vi "get version info.vi"(8 "error in":errorcluster) -> (0 "error out":errorcluster, 2 "FileVersion":string, 3 "Title":string)   [LabVIEW 2023]
doc: "This VI will return the Version info of the exe during runtime environment."
panel:
  in  "Date":string=" Build Date: 09-Jan-2025 "
  # "VI Template By\n        Samuel James\n        Measurement Engineer\n        Certified LabVIEW Architect\n        Vestas Technology R&D Chennai"
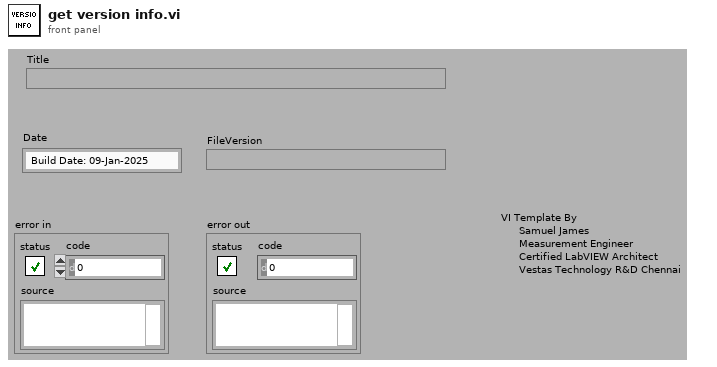
[diagram p1: front panel]
types:
  T1 = enum32{"invalid app kind", "Development System", "Run Time System", "Student Edition", "Embedded LabVIEW", "Evaluation", "Custom"}
  T2 = cluster{"Major":i32, "Minor":i32, "Micro":i32, "Build":i32}
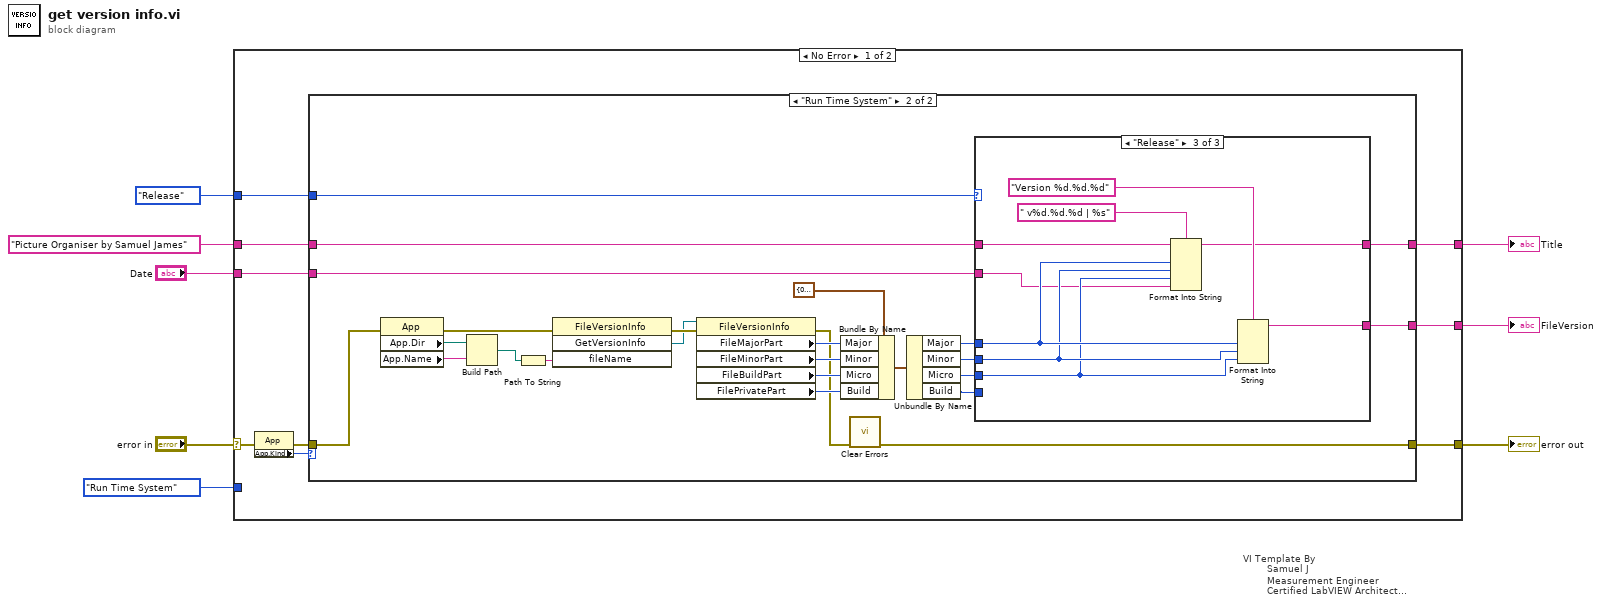
[diagram p0: block diagram]
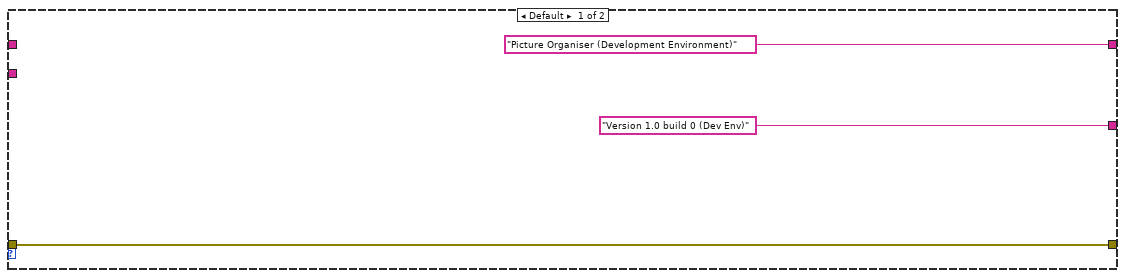
[diagram p2: hidden frame]
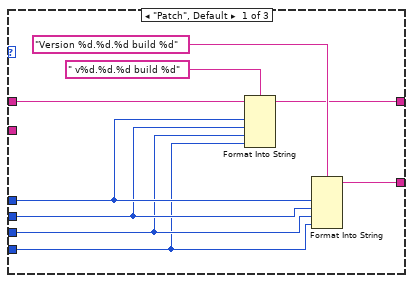
[diagram p3: hidden frame]
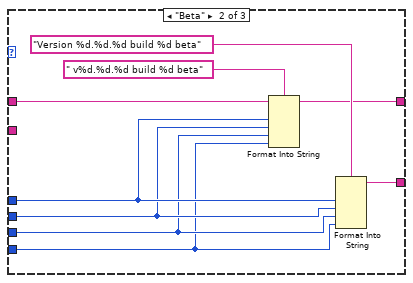
[diagram p4: hidden frame]
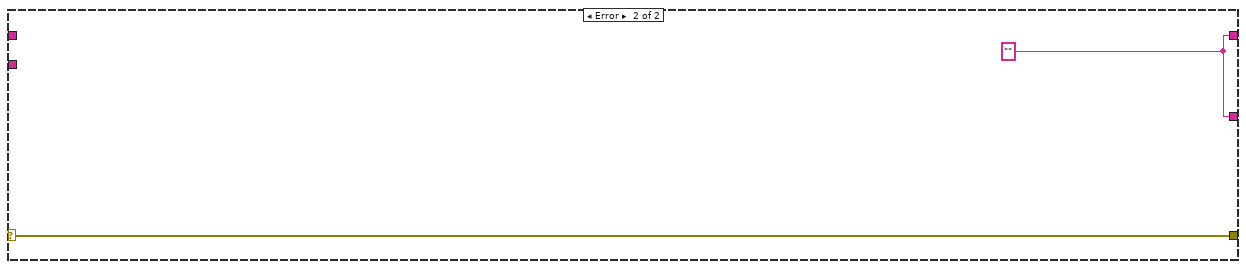
[diagram p5: hidden frame]
diagram:
  n1 = case "VI Template By\n        Samuel J\n        Measurement Engineer\n        Certified LabVIEW Architect\n        Vestas Technology R&D, Chennai" shown="No Error" "error in" {
    selector: "error in" -> [w12 w74]
    tunnel: [w17 w73] -> w8
    tunnel: [w16 w74] -> w6
    tunnel: [w14 w73] -> w5
    tunnel: "Picture Organiser by Samuel James" ("Product Name") -> [w13 _]
    tunnel: T1."Run Time System" ("App.Kind") -> [_ _]
    tunnel: enum16{"Release", "Patch", "Beta"}."Release" -> [w11 _]
    tunnel: "Date" -> [w10 _]
    frame No Error {
      n2 = property class="App"(error in=w12) -> (error out=w15:errorcluster, "App.Kind"=w9:T1)  [unwired: 1 in, 1 out]
      n3 = case shown="\"Run Time System\"" w9 {
        tunnel: ["Version 1.0 build 0 (Dev Env)" w45] -> w17
        tunnel: [w20 w23] -> w16
        tunnel: w15 -> [w20 w42]
        tunnel: ["Picture Organiser (Development Environment)" w44] -> w14
        tunnel: w13 -> [_ w43]
        tunnel: w11 -> [_ w29]
        tunnel: w10 -> [_ w22]
        frame Default {
        }
        frame "Run Time System" {
          n4 = property class="App"(error in=w42) -> (error out=w41:errorcluster, "App.Dir"=w36:path, "App.Name"=w37:string)  [unwired: 1 in, 1 out]
          n5 = Build Path(base path=w36, name or relative path=w37) -> (appended path=w21:path)
          n6 = Path To String(path=w21) -> (string=w40:string)
          n7 = invoke class="FileVersionInfo" method="GetVersionInfo"(error in=w41, "fileName"=w40) -> (error out=w39:errorcluster, "GetVersionInfo"=w38:refnum<k24>)  [unwired: 2 in, 2 out]
          n8 = property class="FileVersionInfo"(reference=w38, error in=w39) -> (error out=w30:errorcluster, "FileMajorPart"=w34:i32, "FileMinorPart"=w33:i32, "FileBuildPart"=w32:i32, "FilePrivatePart"=w31:i32)  [unwired: 1 out]
          n9 = Bundle By Name(cluster=T2 {"Major"=0, "Minor"=0, "Micro"=0, "Build"=0} ("Cluster"), "Major"=w34, "Minor"=w33, "Micro"=w32, "Build"=w31) -> (w28:T2)
          n10 = call <vilib>:"Clear Errors.vi"("error in (no error)"=w30) -> ("error out"=w23:errorcluster)  [unwired: 5 in, 1 out]
          n11 = Unbundle By Name(w28) -> ("Major"=w27:i32, "Minor"=w26:i32, "Micro"=w25:i32, "Build"=w24:i32)
          n12 = case shown="\"Release\"" w29 {
            tunnel: [w53 w62 w71] -> w45
            tunnel: [w51 w60 w69] -> w44
            tunnel: w43 -> [w50 w59 w68]
            tunnel: w27 -> [w49 w58 w67]
            tunnel: w26 -> [w48 w57 w66]
            tunnel: w25 -> [w47 w56 w65]
            tunnel: w24 -> [w46 w55 _]
            tunnel: w22 -> [_ _ w64]
            frame "Patch", Default {
              n13 = Format Into String(format string=" v%d.%d.%d build %d", initial string=w50, w49, w48, w47, w46) -> (resulting string=w51:string)  [unwired: 1 in, 1 out]
              n14 = Format Into String(format string="Version %d.%d.%d build %d", w49, w48, w47, w46) -> (resulting string=w53:string)  [unwired: 2 in, 1 out]
            }
            frame "Beta" {
              n15 = Format Into String(format string=" v%d.%d.%d build %d beta", initial string=w59, w58, w57, w56, w55) -> (resulting string=w60:string)  [unwired: 1 in, 1 out]
              n16 = Format Into String(format string="Version %d.%d.%d build %d beta", w58, w57, w56, w55) -> (resulting string=w62:string)  [unwired: 2 in, 1 out]
            }
            frame "Release" {
              n17 = Format Into String(format string=" v%d.%d.%d | %s", initial string=w68, w67, w66, w65, w64) -> (resulting string=w69:string)  [unwired: 1 in, 1 out]
              n18 = Format Into String(format string="Version %d.%d.%d", w67, w66, w65) -> (resulting string=w71:string)  [unwired: 2 in, 1 out]
            }
          }
        }
      }
    }
    frame Error {
      w73 = ""
    }
  }
  "FileVersion" <- w8
  "error out" <- w6
  "Title" <- w5
